vi "筛选相同用户名通道.vi"(10 "通道in":string[][](array[string])) -> (2 "通道":string[][](array[string]))   [LabVIEW 2015]
uses:
  Global/Globalclient.vi
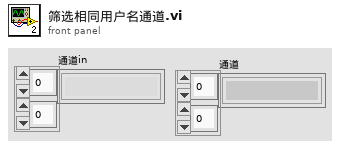
[diagram p1: front panel]
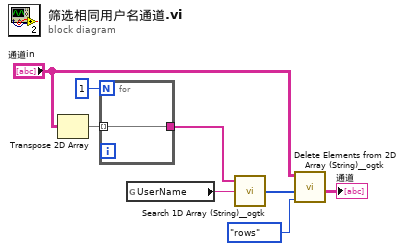
[diagram p0: block diagram]
diagram:
  n1 = Transpose 2D Array(2D array="通道in") -> (transposed array=w8:string[][])
  n2 = for {
    N: 1 -> [_]
    tunnel: w8 -> [w9] mode=indexing
    tunnel: [w9] -> w6
  }
  n3 = global read "Globalclient.vi" "UserName"() -> (w5:string)
  n4 = call <userlib>:"Search 1D Array (String)__ogtk.vi"("Array"=w6, "Element Data"=w5) -> ("Indices of Elements"=w4:i32[])  [unwired: 7 in]
  n5 = call <userlib>:"Delete Elements from 2D Array (String)__ogtk.vi"("delete (rows or columns)"=enum16{"rows", "columns"}."rows", "indices"=w4, "array"="通道in") -> ("deleted elements"=→"通道":string[][])  [unwired: 7 in, 1 out]
